vi "reset AO_DO.vi"() -> ()   [LabVIEW 2015]
uses:
  <vilib>/DAQmx/write.llb/DAQmx Write.vi
  <vilib>/DAQmx/write.llb/DAQmx Write (Digital 1D Bool NChan 1Samp 1Line).vi
  <vilib>/DAQmx/write.llb/DAQmx Write (Analog 1D DBL NChan 1Samp).vi
  <vilib>/DAQmx/create/channels.llb/DAQmx Create Channel (DO-Digital Output).vi
  <vilib>/DAQmx/miscellaneous.llb/DAQmx Fill In Error Info.vi
  <vilib>/DAQmx/create/channels.llb/DAQmx Create Channel (AO-Voltage-Basic).vi
  <resource>/objmgr/daqmx.rc
panel:
  in  "error in 2":errorcluster caption="error in"
  in  "error in":errorcluster
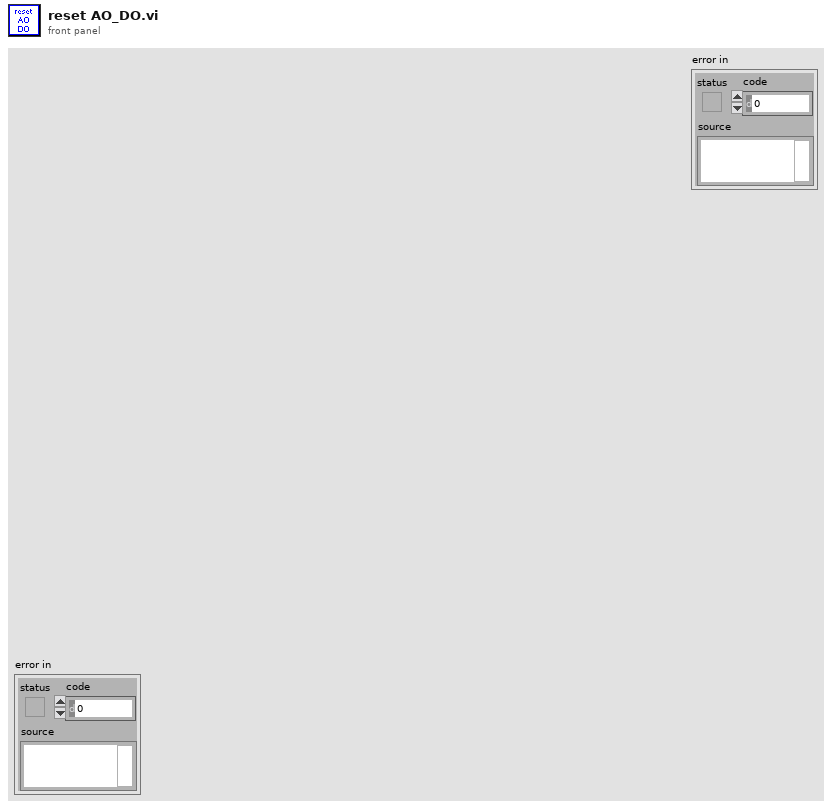
[diagram p1: front panel]
types:
  T1 = cluster{"StageS":i32, "StageL":i32, "currmeas data dir":path, "image OD":u16, "contour OD":u16, "point OD":u16, "AOlines":tag[], "AIlines":tag[], "CI lines":tag[], "DO lines":tag[], "AO names":string[], "CI names":string[], "AI names":string[], "DO names":string[], "CIextensions":string[], "AIextensions":string[], "Voltage to Ygalvo":i32, "Voltage to Xgalvo":i32, "Voltage to patch":i32, "640 shutter":i32, "2P shutter":i32, "LT timestamp":u32, "Vp":i32, "Ip":i32, "camera trigger":i32, "master data dir":path}
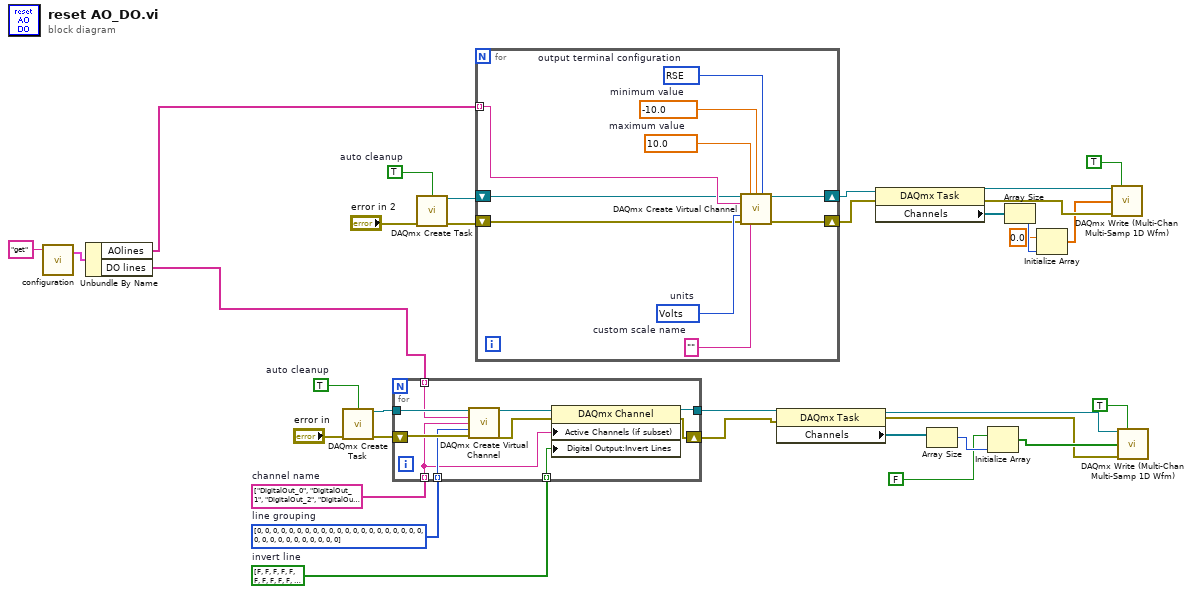
[diagram p0: block diagram]
diagram:
  w14 = TRUE  # auto cleanup
  w30 = bool[] [FALSE, FALSE, FALSE, FALSE, FALSE, FALSE, FALSE, FALSE, FALSE, FALSE, FALSE, FALSE, FALSE, FALSE, FALSE, FALSE, FALSE, FALSE, FALSE, FALSE, FALSE, FALSE, FALSE, FALSE, FALSE, FALSE, FALSE, FALSE, FALSE, FALSE, FALSE, FALSE]  # invert line
  w31 = i32[] [0, 0, 0, 0, 0, 0, 0, 0, 0, 0, 0, 0, 0, 0, 0, 0, 0, 0, 0, 0, 0, 0, 0, 0, 0, 0, 0, 0, 0, 0, 0, 0] items=["one channel for each line", "one channel for all lines"]  # line grouping
  w32 = string[] ["DigitalOut_0", "DigitalOut_1", "DigitalOut_2", "DigitalOut_3", "DigitalOut_4", "DigitalOut_5", "DigitalOut_6", "DigitalOut_7", "DigitalOut_8", "DigitalOut_9", "DigitalOut_10", "DigitalOut_11", "DigitalOut_12", "DigitalOut_13", "DigitalOut_14", "DigitalOut_15", "DigitalOut_16", "DigitalOut_17", "DigitalOut_18", "DigitalOut_19", "DigitalOut_20", "DigitalOut_21", "DigitalOut_22", "DigitalOut_23", "DigitalOut_24", "DigitalOut_25", "DigitalOut_26", "DigitalOut_27", "DigitalOut_28", "DigitalOut_29", "DigitalOut_30", "DigitalOut_31"]  # channel name
  w28 = TRUE  # auto cleanup
  n1 = call "configuration.vi"("command"="get") -> ("config out"=w3:T1)  [unwired: 2 in, 1 out]
  n2 = Unbundle By Name(w3) -> ("AOlines"=w2:tag[], "DO lines"=w1:tag[])
  n3 = call <vilib>:"DAQmx Create Task.vi"("auto cleanup"=w28, "error in"="error in") -> ("task out"=w29:refnum<k21>, "error out"=w27:errorcluster)  [unwired: 12 in]
  n4 = for {
    tunnel: w29 -> [w43]
    tunnel: w30 -> [w37] mode=indexing
    tunnel: w31 -> [w40] mode=indexing
    tunnel: w32 -> [w36] mode=indexing
    tunnel: w1 -> [w41] mode=indexing
    tunnel: [w38] -> w23
    shift-right: [w34] -> w22
    shift-left: w27 -> [w42]
    n5 = call-poly <vilib>:"DAQmx Create Virtual Channel.vi"("task in"=w43, "lines"=w41, "name to assign"=w36, "line grouping"=w40, "error in"=w42) -> ("task out"=w39:refnum<k21>, "error out"=w35:errorcluster)  [unwired: 9 in]
    n6 = property class="DAQmx Channel"(reference=w39, error in=w35, "Active Channels (if subset)"=w36, "Digital Output:Invert Lines"=w37) -> (reference out=w38:refnum<k21>, error out=w34:errorcluster)
  }
  n7 = call <vilib>:"DAQmx Create Task.vi"("auto cleanup"=w14, "error in"="error in 2") -> ("task out"=w15:refnum<k21>, "error out"=w16:errorcluster)  [unwired: 12 in]
  n8 = for {
    tunnel: w2 -> [w48] mode=indexing
    shift-right: [w45] -> w11
    shift-left: w15 -> [w47]
    shift-right: [w44] -> w10
    shift-left: w16 -> [w46]
    w53 = 10083 items=["Default"=-1, "RSE"=10083, "Differential"=10106, "Pseudodifferential"=12529]  # output terminal configuration
    w52 = 10348 items=["Volts"=10348, "From Custom Scale"=10065]  # units
    w51 = ""  # custom scale name
    w50 = -10.0  # minimum value
    w49 = 10.0  # maximum value
    n9 = call-poly <vilib>:"DAQmx Create Virtual Channel.vi"("task in"=w47, "maximum value"=w49, "minimum value"=w50, "output terminal configuration"=w53, "physical channels"=w48, "units"=w52, "error in"=w46, "custom scale name"=w51) -> ("task out"=w45:refnum<k21>, "error out"=w44:errorcluster)  [unwired: 6 in]
  }
  n10 = property class="DAQmx Task"(reference=w23, error in=w22) -> (reference out=w19:refnum<k21>, error out=w18:errorcluster, "Channels"=w24:refnum<k21>[])
  n11 = property class="DAQmx Task"(reference=w11, error in=w10) -> (reference out=w7:refnum<k21>, error out=w8:errorcluster, "Channels"=w12:refnum<k21>[])
  n12 = Array Size(array=w24) -> (size(s)=w25:i32)
  n13 = Initialize Array(FALSE ("initial value"), w25) -> (w20:bool[])
  n14 = Array Size(array=w12) -> (size(s)=w6:i32)
  n15 = Initialize Array(0.0 ("element"), w6) -> (w4:dbl[])
  n16 = call-poly "DAQmx Write (Multi-Chan Multi-Samp 1D Wfm).vi"("task/channels in"=w7, "auto start"=TRUE, "data"=w4, "error in"=w8) -> ()  [unwired: 9 in, 3 out]
  n17 = call-poly "DAQmx Write (Multi-Chan Multi-Samp 1D Wfm).vi"("task/channels in"=w19, "auto start"=TRUE, "data"=w20, "error in"=w18) -> ()  [unwired: 9 in, 3 out]
